vi "Actor Core.vi"(8 "error in":errorcluster, 11 "CoolAppProcess in":refnum<class "CoolAppProcess.lvclass">) -> (0 "error out":errorcluster, 3 "Actor out":refnum<class "Actor.lvclass">)   [LabVIEW 2020, in "LAF2024Q2.lvlib" / "CoolAppProcess.lvclass"]
doc: "(<B>Filename</B>: Actor Framework.lvlib:Actor.lvclass:Actor Core.vi)\n\nReceives messages to the actor, reacts to them, and initiates any error handling that may shut the actor down.\n\nDescendant classes may override this VI to append parallel tasks for the actor to complete while it handles messages. Overrides use the Call Parent Class Method node."
uses:
  CoolAppProcess.lvclass
  C:/Program Files (x86)/National Instruments/LabVIEW 2020/vi.lib/ActorFramework/Actor/Actor.lvclass
  <vilib>/ActorFramework/Actor/Actor.lvclass
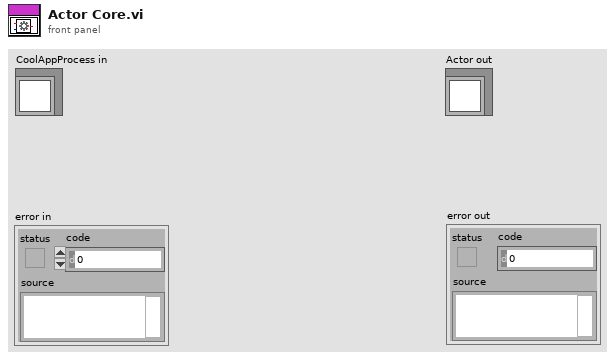
[diagram p1: front panel]
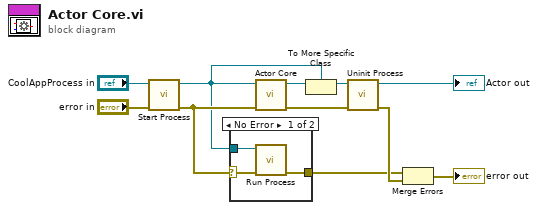
[diagram p0: block diagram]
diagram:
  n1 = call-dynamic "Start Process.vi"("error in (no error)"="error in", "CoolAppProcess in"="CoolAppProcess in") -> ("error out"=w3:errorcluster, "CoolAppProcess out"=w2:refnum<class "CoolAppProcess.lvclass">)  [unwired: 8 in]
  n2 = case shown="No Error" w3 {
    selector: w3 -> [w14 _]
    tunnel: w2 -> [w13 _]
    tunnel: [w12 _] -> w1
    frame No Error {
      n3 = call-dynamic "Run Process.vi"("error in (no error)"=w14, "CoolAppProcess in"=w13) -> ("error out"=w12:errorcluster)  [unwired: 8 in, 1 out]
    }
    frame Error {
    }
  }
  n4 = call-parent "Actor Core.vi"("error in"=w3, "Actor in"=w2) -> ("error out"=w10:errorcluster, "Actor out"=w9:refnum<class "Actor.lvclass">)  [unwired: 8 in]
  n5 = To More Specific Class(target class=w2, reference=w9) -> (specific class reference=w7:refnum<class "CoolAppProcess.lvclass">)  [unwired: 1 in, 1 out]
  n6 = call-dynamic "Uninit Process.vi"("error in (no error)"=w10, "CoolAppProcess in"=w7) -> ("error out"=w8:errorcluster, "CoolAppProcess out"=→"Actor out":refnum<class "CoolAppProcess.lvclass">)  [unwired: 8 in]
  n7 = Merge Errors(w1, w8) -> (→"error out":errorcluster)
